vi "素材.vi"() -> ()   [LabVIEW 2018]
uses:
  <vilib>/Analysis/4window.llb/Hanning Window (DBL).vi
  <vilib>/Analysis/2dsp.llb/Real FFT.vi
  <vilib>/Analysis/4window.llb/AllCosWindow (DBL).vi
  <vilib>/Analysis/NI_AALBase.lvlib
  <vilib>/Analysis/NI_AALPro.lvlib
panel:
  out "波形图 3":dbl[](graph)
  out "波形图 2":dbl[](graph)
  out "波形图":dbl[][](graph)
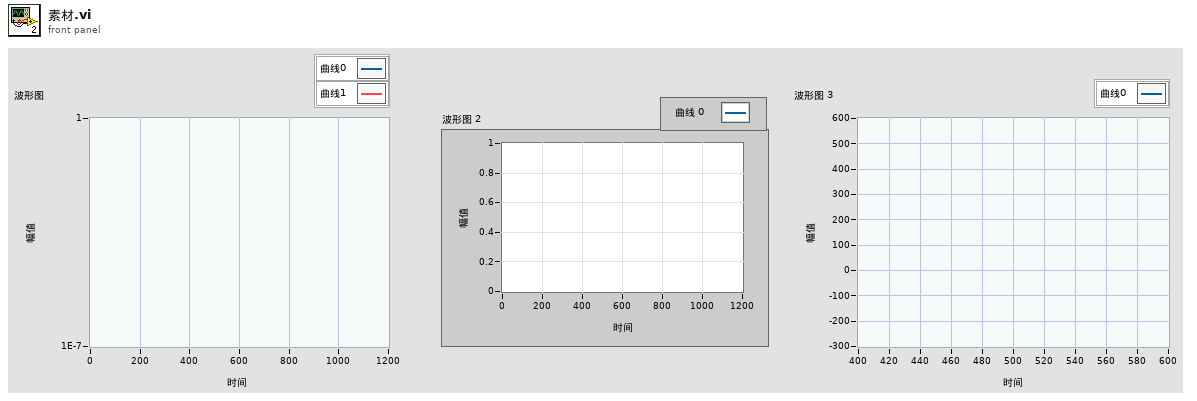
[diagram p1: front panel]
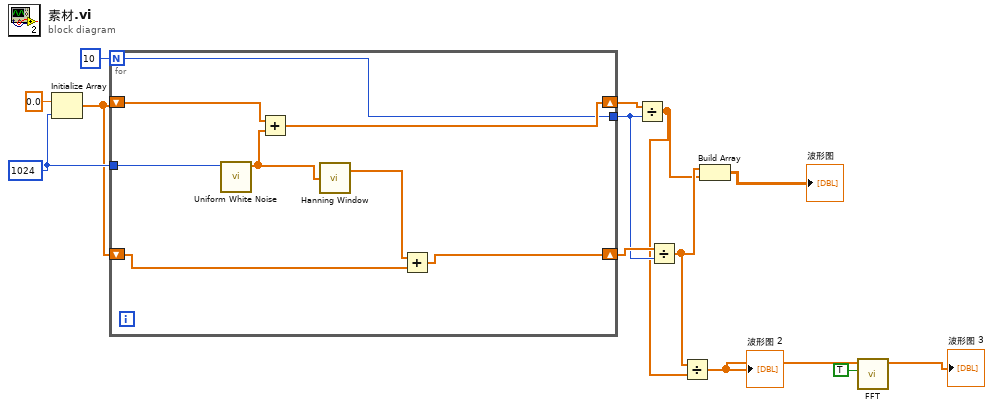
[diagram p0: block diagram]
diagram:
  w11 = 1024 ("samples")
  n1 = Initialize Array(0.0 ("元素"), w11) -> (w9:dbl[])
  n2 = for {
    N: 10 -> [w17]
    tunnel: w11 -> [w21]
    shift-right: [w18] -> w10
    shift-left: w9 -> [w19]
    tunnel: [w17] -> w7
    shift-right: [w14] -> w8
    shift-left: w9 -> [w16]
    n3 = call <vilib>:"Uniform White Noise.vi"("samples"=w21) -> ("uniform white noise"=w20:dbl[])  [unwired: 9 in, 1 out]
    n4 = Add(x=w19, y=w20) -> (x+y=w18:dbl[])
    n5 = call-poly <vilib>:"Hanning Window.vi"("X"=w20) -> ("Windowed X"=w15:dbl[])  [unwired: 1 out]
    n6 = Add(x=w15, y=w16) -> (x+y=w14:dbl[])
  }
  n7 = Divide(x=w10, y=w7) -> (x/y=w4:dbl[])
  n8 = Divide(x=w8, y=w7) -> (x/y=w5:dbl[])
  n9 = Divide(x=w5, y=w4) -> (x/y=w3:dbl[])
  "波形图 2" <- w3
  n10 = Build Array(w5, w4) -> (→"波形图":dbl[][])
  n11 = call-poly <vilib>:"FFT.vi"("shift?"=TRUE, "X"=w3) -> ("FFT {X}"=→"波形图 3":cdb[])  [unwired: 8 in, 1 out]
